vi "get default message.vi"(11 "exception in":T1 {"code" format="%.0x"}) -> (2 "message":string, 3 "exception out":T1 {"code" format="%.0x"})   [LabVIEW 2013, in "exception.lvlib"]
uses:
  exception.lvlib
  exception.ctl
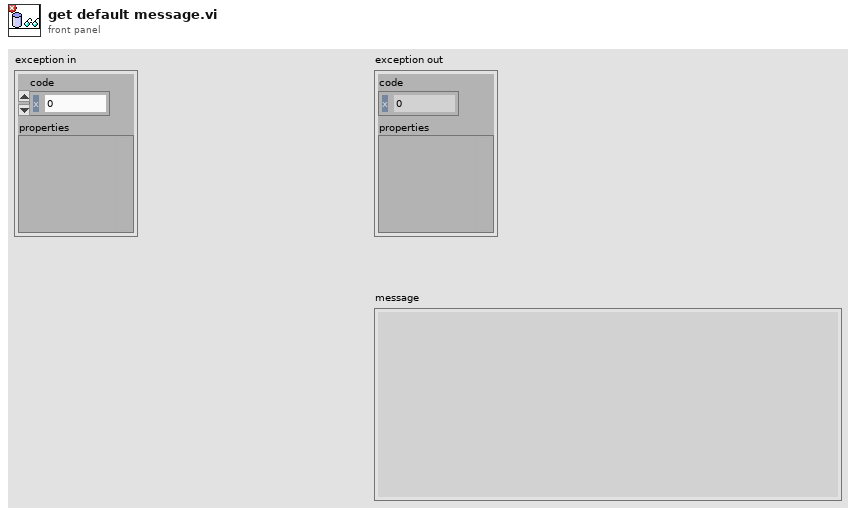
[diagram p1: front panel]
types:
  T1 = typedef "exception.lvlib/exception.ctl" = cluster{"code":i32, "properties":variant}
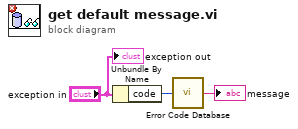
[diagram p0: block diagram]
diagram:
  n1 = Unbundle By Name("exception in") -> ("code"=w2:i32)
  n2 = call <vilib>:"Error Code Database.vi"("Error Code"=w2) -> ("Error Text"=→"message":string)
  "exception out" <- "exception in"
